vi "SetupAquisitionParameters.vi"(5 "error in":errorcluster) -> (19 "error out":errorcluster)   [LabVIEW 2010]
uses:
  lib/atmcd32d.llb/Error Code Enum typedef.ctl
  lib/atmcd32d.llb/AcquisitionMode_mode typedef.ctl
  lib/atmcd32d.llb/TriggerMode_mode typedef.ctl
  lib/atmcd32d.llb/ReadMode_mode typedef.ctl
  lib/atmcd32d.llb/OutputAmplifier_type typedef.ctl
  lib/atmcd32d.llb/Spool_method typedef.ctl
  Variables/GlobalGetSetMeasurementType.vi
  Variables/GlobalSetGetConfigureCamera.vi
  Variables/GlobalSetGetPixelOfRoi.vi
  Variables/GlobalGetTimingsFromCamera.vi
  lib/atmcd32d.llb/Shutter_mode typedef.ctl
  lib/atmcd32d.llb/Shutter_type typedef.ctl
  lib/atmcd32d.llb/EMGainMode_mode typedef.ctl
panel:
  out "keepCleanTime":sgl
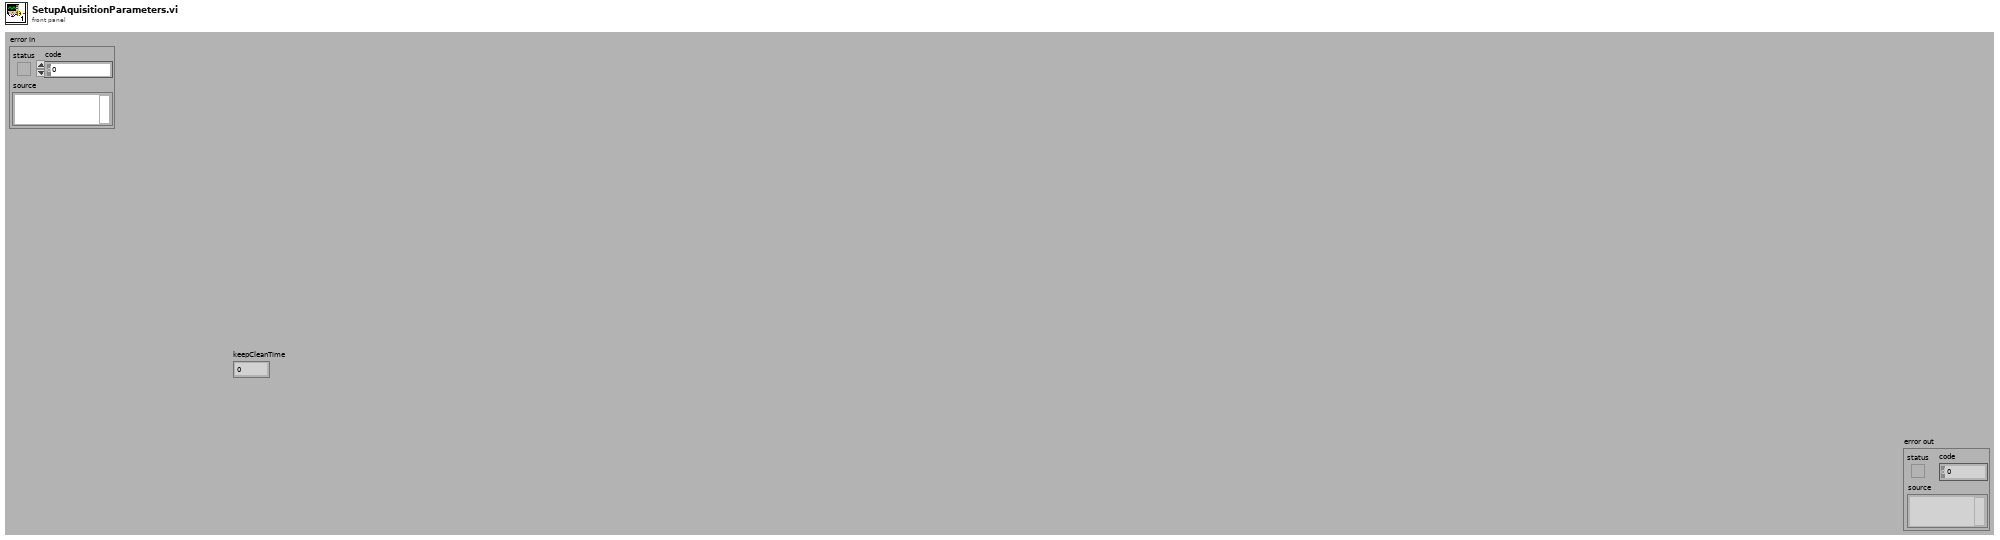
[diagram p1: front panel]
types:
  T1 = cluster{"exposure":sgl, "accumulate":sgl, "kinetic":sgl}
  T2 = typedef "Error Code Enum typedef.ctl" = enum32{"N/A (0)", "DRV_ERROR_CODES", "DRV_SUCCESS", "DRV_VXDNOTINSTALLED", "DRV_ERROR_SCAN", "DRV_ERROR_CHECK_SUM", "DRV_ERROR_FILELOAD", "DRV_UNKNOWN_FUNC", "DRV_ERROR_VXD_INIT", "DRV_ERROR_ADDRESS", "DRV_ERROR_PAGELOCK", "DRV_ERROR_PAGEUNLOCK", "DRV_ERROR_BOARDTEST", "DRV_ERROR_ACK", "DRV_ERROR_UP_FIFO", "DRV_ERROR_PATTERN", "N/A (16)", "DRV_ACQUISITION_ERRORS", "DRV_ACQ_BUFFER", "DRV_ACQ_DOWNFIFO_FULL", "DRV_PROC_UNKONWN_INSTRUCTION", "DRV_ILLEGAL_OP_CODE", "DRV_KINETIC_TIME_NOT_MET", "DRV_ACCUM_TIME_NOT_MET", "DRV_NO_NEW_DATA", "N/A (25)", "DRV_SPOOLERROR", "N/A (27)", "N/A (28)", "N/A (29)", "N/A (30)", "N/A (31)", "N/A (32)", "DRV_TEMPERATURE_CODES", "DRV_TEMPERATURE_OFF", "DRV_TEMPERATURE_NOT_STABILIZED", "DRV_TEMPERATURE_STABILIZED", "DRV_TEMPERATURE_NOT_REACHED", "DRV_TEMPERATURE_OUT_RANGE", "DRV_TEMPERATURE_NOT_SUPPORTED", "DRV_TEMPERATURE_DRIFT", "N/A (41)", "N/A (42)", "N/A (43)", "N/A (44)", "N/A (45)", "N/A (46)", "N/A (47)", "N/A (48)", "DRV_GENERAL_ERRORS", "DRV_INVALID_AUX", "DRV_COF_NOTLOADED", "DRV_FPGAPROG", "DRV_FLEXERROR", "DRV_GPIBERROR", "N/A (55)", "N/A (56)", "N/A (57)", "N/A (58)", "N/A (59)", "N/A (60)", "N/A (61)", "N/A (62)", "N/A (63)", "DRV_DATATYPE", "DRV_DRIVER_ERRORS", "DRV_P1INVALID", "DRV_P2INVALID", "DRV_P3INVALID", "DRV_P4INVALID", "DRV_INIERROR", "DRV_COFERROR", "DRV_ACQUIRING", "DRV_IDLE", "DRV_TEMPCYCLE", "DRV_NOT_INITIALIZED", "DRV_P5INVALID", "DRV_P6INVALID", "DRV_INVALID_MODE", "DRV_INVALID_FILTER", "DRV_I2CERRORS", "DRV_I2CDEVNOTFOUND", "DRV_I2CTIMEOUT", "DRV_P7INVALID", "N/A (84)", "N/A (85)", "N/A (86)", "N/A (87)", "N/A (88)", "N/A (89)", "DRV_IOCERROR", "DRV_VRMVERSIONERROR"}
  T3 = typedef "EMGainMode_mode typedef.ctl" = enum16{"8-bit", "12-bit", "Linear", "Real"}
  T4 = typedef "AcquisitionMode_mode typedef.ctl" = enum16{"Reserved (0)", "Single Scan", "Accumulate", "Kinetics", "Fast Kinetics", "Run Till Abort", "Reserved (6)", "Reserved (7)", "Reserved (8)", "Time Delayed Integration"}
  T5 = typedef "Spool_method typedef.ctl" = enum16{"32-bit", "Depends", "16-bit", "Multiple Directory", "Spool to RAM disk", "16-bit FITS", "SIF", "16-buit TIFF", "Multiple Directory Compressed"}
  T6 = typedef "OutputAmplifier_type typedef.ctl" = enum16{"Standard EMCCD gain register", "Conventional CCD register"}
  T7 = typedef "ReadMode_mode typedef.ctl" = enum16{"Full Vertical Binning", "Multi-Track", "Random-Track", "Single-Track", "Image"}
  T8 = typedef "TriggerMode_mode typedef.ctl" = enum16{"Internal", "External", "N/A (2)", "N/A (3)", "N/A (4)", "N/A (5)", "External Start"}
  T9 = typedef "Shutter_type typedef.ctl" = enum16{"TTL Low", "TTL High"}
  T10 = typedef "Shutter_mode typedef.ctl" = enum16{"Auto", "Open", "Close"}
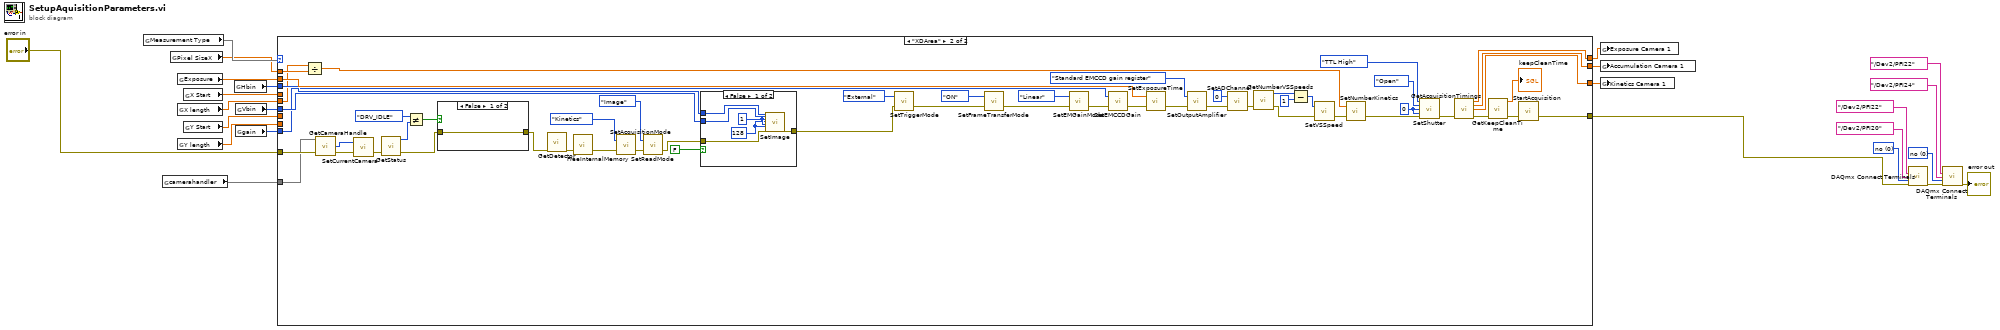
[diagram p0: block diagram]
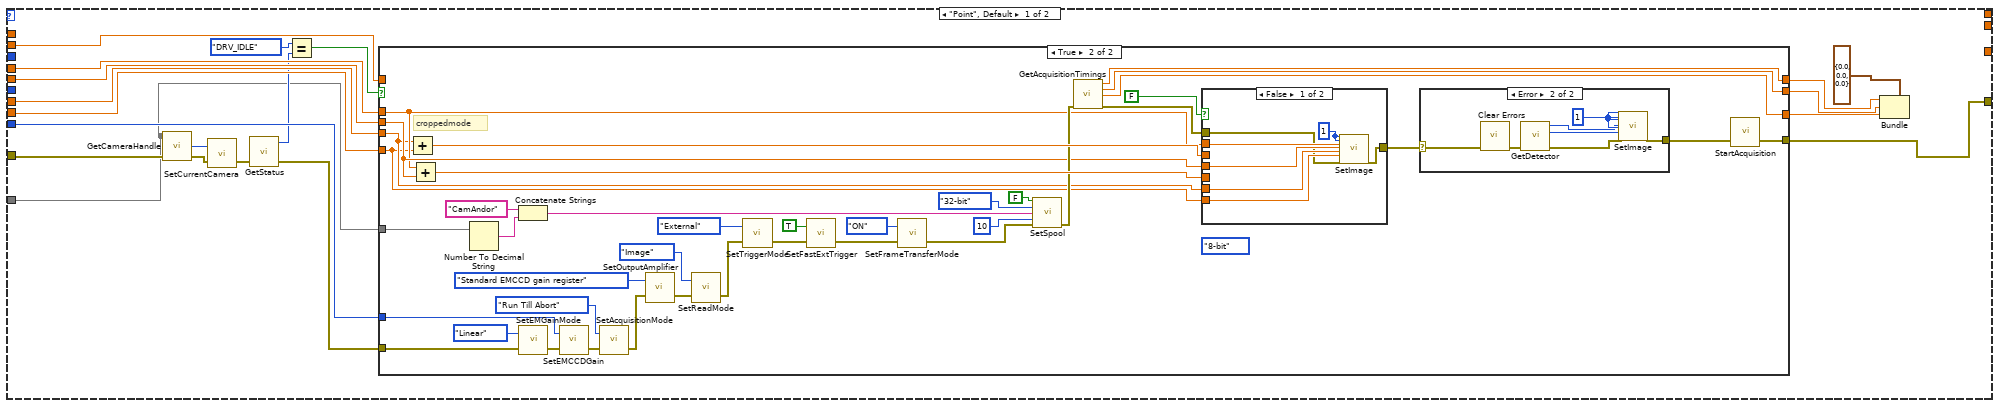
[diagram p2: hidden frame]
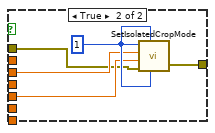
[diagram p4: hidden frame]
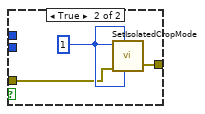
[diagram p6: hidden frame]
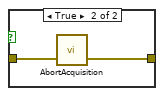
[diagram p7: hidden frame]
diagram:
  w24 = 0 items=["no", "yes"] ("invert polarity")
  w20 = 0 items=["no", "yes"] ("invert polarity")
  n1 = global read "GlobalGetSetMeasurementType.vi" "Measurement Type"() -> (w14)
  n2 = global read "GlobalSetGetConfigureCamera.vi" "camerahandler"() -> (w1)
  n3 = global read "GlobalSetGetPixelOfRoi.vi" "Pixel SizeX"() -> (w10:dbl)
  n4 = global read "GlobalSetGetConfigureCamera.vi" "Exposure"() -> (w13:sgl)
  n5 = global read "GlobalSetGetPixelOfRoi.vi" "X length"() -> (w9:dbl)
  n6 = global read "GlobalSetGetPixelOfRoi.vi" "Y length"() -> (w6:dbl)
  n7 = global read "GlobalSetGetPixelOfRoi.vi" "X Start"() -> (w8:dbl)
  n8 = global read "GlobalSetGetPixelOfRoi.vi" "Y Start"() -> (w7:dbl)
  n9 = global read "GlobalSetGetConfigureCamera.vi" "Hbin"() -> (w11:i32)
  n10 = global read "GlobalSetGetConfigureCamera.vi" "Vbin"() -> (w12:i32)
  n11 = global read "GlobalSetGetConfigureCamera.vi" "gain"() -> (w4:i32)
  n12 = case shown="\"XDArea\"" w14 {
    tunnel: "error in" -> [w44 w158]
    tunnel: w13 -> [w43 w156]
    tunnel: [w42 w157] -> w16
    tunnel: w11 -> [_ w155]
    tunnel: w12 -> [_ w154]
    tunnel: w10 -> [_ w153]
    tunnel: w9 -> [w41 w152]
    tunnel: w8 -> [w40 _]
    tunnel: w7 -> [w39 _]
    tunnel: w6 -> [w38 _]
    tunnel: [_ w108] -> w5
    tunnel: w4 -> [w37 w151]
    tunnel: [_ w107] -> w3
    tunnel: [_ w106] -> w2
    tunnel: w1 -> [w25 w105]
    frame "Point", Default {
      n13 = call "GetCameraHandle.vi"("error in (no error)"=w44, "cameraIndex"=w25) -> ("error out"=w35:errorcluster, "cameraHandle"=w36:i32)  [unwired: 1 in, 1 out]
      n14 = call "SetCurrentCamera.vi"("error in (no error)"=w35, "cameraHandle"=w36) -> ("error out"=w34:errorcluster)  [unwired: 1 out]
      n15 = call "GetStatus.vi"("error in (no error)"=w34) -> ("error out"=w33:errorcluster, "status"=w31:T2)  [unwired: 2 in, 1 out]
      n16 = Equal?(x=Error_Code_Enum_typedef."DRV_IDLE" ("status"), y=w31) -> (x = y?=w30:bool)
      n17 = case shown="True" w30 {
        tunnel: [w45 w81] -> w42
        tunnel: w33 -> [w45 w46]
        tunnel: w25 -> [_ w78]
        tunnel: w43 -> [_ _]
        tunnel: [_ w69] -> w29
        tunnel: [_ w68] -> w28
        tunnel: [_ w67] -> w27
        tunnel: w41 -> [_ w55]
        tunnel: w40 -> [_ w54]
        tunnel: w39 -> [_ w53]
        tunnel: w38 -> [_ w52]
        tunnel: w37 -> [_ w47]
        frame False {
        }
        frame True {
          (unwired) EMGainMode_mode_typedef."8-bit" ("mode")
          # "croppedmode"
          n18 = Add(x=w53, y=w52) -> (x+y=w74:dbl)
          n19 = Add(x=w54, y=w55) -> (x+y=w73:dbl)
          n20 = Number To Decimal String(number=w78) -> (decimal integer string=w79:string)  [unwired: 1 in]
          n21 = Concatenate Strings("CamAndor" ("string"), w79) -> (w77:string)
          n22 = call "SetEMGainMode.vi"("error in (no error)"=w46, "mode"=EMGainMode_mode_typedef."Linear") -> ("error out"=w50:errorcluster)  [unwired: 1 out]
          n23 = call "SetEMCCDGain.vi"("error in (no error)"=w50, "gain"=w47) -> ("error out"=w49:errorcluster)  [unwired: 1 out]
          n24 = call "SetAcquisitionMode.vi"("error in (no error)"=w49, "mode"=AcquisitionMode_mode_typedef."Run Till Abort") -> ("error out"=w76:errorcluster)  [unwired: 1 out]
          n25 = call "SetOutputAmplifier.vi"("error in (no error)"=w76, "type"=OutputAmplifier_type_typedef."Standard EMCCD gain register") -> ("error out"=w56:errorcluster)  [unwired: 1 out]
          n26 = call "SetReadMode.vi"("error in (no error)"=w56, "mode"=ReadMode_mode_typedef."Image") -> ("error out"=w83:errorcluster)  [unwired: 1 out]
          n27 = call "SetTriggerMode.vi"("error in (no error)"=w83, "mode"=TriggerMode_mode_typedef."External") -> ("error out"=w82:errorcluster)  [unwired: 1 out]
          n28 = call "SetFastExtTrigger.vi"("error in (no error)"=w82, "mode"=TRUE) -> ("error out"=w84:errorcluster)  [unwired: 1 out]
          n29 = call "SetFrameTransferMode.vi"("error in (no error)"=w84, "mode"=enum16{"OFF", "ON"}."ON") -> ("error out"=w51:errorcluster)  [unwired: 1 out]
          n30 = call "SetSpool.vi"("active"=FALSE, "method"=Spool_method_typedef."32-bit", "name"=w77, "framebuffersize (10)"=10, "error in (no error)"=w51) -> ("error out"=w70:errorcluster)  [unwired: 9 in, 1 out]
          n31 = call "GetAcquisitionTimings.vi"("error in (no error)"=w70) -> ("exposure"=w69:sgl, "accumulate"=w68:sgl, "kinetic"=w67:sgl, "error out"=w72:errorcluster)  [unwired: 10 in, 1 out]
          n32 = case shown="False" FALSE {
            tunnel: w74 -> [_ w95]
            tunnel: w73 -> [_ w94]
            tunnel: w72 -> [w87 w93]
            tunnel: [w86 w92] -> w71
            tunnel: w54 -> [w90 _]
            tunnel: w53 -> [w89 _]
            tunnel: w55 -> [w91 _]
            tunnel: w52 -> [w88 _]
            frame False {
              w85 = 1
              n33 = call "SetImage.vi"("hbin"=w85, "vbin"=w85, "hstart"=w90, "hend"=w91, "vstart"=w89, "vend"=w88, "error in (no error)"=w87) -> ("error out"=w86:errorcluster)  [unwired: 19 in, 1 out]
            }
            frame True {
              w96 = 1 ("hbin")
              n34 = call "SetIsolatedCropMode.vi"("hbin"=w96, "vbin"=w96, "error in (no error)"=w93, "cropWidth"=w94, "cropHeight"=w95, "active"=w96) -> ("error out"=w92:errorcluster)  [unwired: 1 out]
            }
          }
          n35 = case shown="Error" w71 {
            selector: w71 -> [w97 w100]
            tunnel: [w97 w104] -> w75
            frame No Error {
            }
            frame Error {
              w103 = 1
              n36 = call <vilib>:"Clear Errors.vi"("error in (no error)"=w100) -> ("error out"=w101:errorcluster)  [unwired: 6 in]
              n37 = call "GetDetector.vi"("error in (no error)"=w101) -> ("error out"=w102:errorcluster, "ypixels"=w98:i32, "xpixels"=w99:i32)  [unwired: 3 in, 1 out]
              n38 = call "SetImage.vi"("hbin"=w103, "vbin"=w103, "hstart"=w103, "hend"=w99, "vstart"=w103, "vend"=w98, "error in (no error)"=w102) -> ("error out"=w104:errorcluster)  [unwired: 19 in, 1 out]
            }
          }
          n39 = call "StartAcquisition.vi"("error in (no error)"=w75) -> ("error out"=w81:errorcluster)  [unwired: 1 in, 1 out]
        }
      }
      n40 = Bundle(cluster=T1 {"exposure"=0.0, "accumulate"=0.0, "kinetic"=0.0} ("out 2"), "exposure"=w29, "accumulate"=w28, "kinetic"=w27) -> ()  [unwired: 1 out]
    }
    frame "XDArea" {
      w117 = 0 ("closingtime")
      n41 = Divide(x=w152, y=w153) -> (x/y=w136:dbl)
      n42 = call "GetCameraHandle.vi"("error in (no error)"=w158, "cameraIndex"=w105) -> ("error out"=w149:errorcluster, "cameraHandle"=w150:i32)  [unwired: 1 in, 1 out]
      n43 = call "SetCurrentCamera.vi"("error in (no error)"=w149, "cameraHandle"=w150) -> ("error out"=w148:errorcluster)  [unwired: 1 out]
      n44 = call "GetStatus.vi"("error in (no error)"=w148) -> ("error out"=w147:errorcluster, "status"=w145:T2)  [unwired: 2 in, 1 out]
      n45 = Not Equal?(x=Error_Code_Enum_typedef."DRV_IDLE" ("status"), y=w145) -> (x != y?=w144:bool)
      n46 = case shown="False" w144 {
        tunnel: w147 -> [w168 w170]
        tunnel: [w168 w169] -> w134
        frame False {
        }
        frame True {
          n47 = call "AbortAcquisition.vi"("error in (no error)"=w170) -> ("error out"=w169:errorcluster)  [unwired: 1 in, 1 out]
        }
      }
      n48 = call "GetDetector.vi"("error in (no error)"=w134) -> ("error out"=w135:errorcluster)  [unwired: 3 in, 3 out]
      n49 = call "FreeInternalMemory.vi"("error in (no error)"=w135) -> ("error out"=w137:errorcluster)  [unwired: 1 in, 1 out]
      n50 = call "SetAcquisitionMode.vi"("error in (no error)"=w137, "mode"=AcquisitionMode_mode_typedef."Kinetics") -> ("error out"=w133:errorcluster)  [unwired: 1 out]
      n51 = call "SetReadMode.vi"("error in (no error)"=w133, "mode"=ReadMode_mode_typedef."Image") -> ("error out"=w132:errorcluster)  [unwired: 1 out]
      n52 = case shown="False" FALSE {
        tunnel: w132 -> [w164 w166]
        tunnel: [w163 w165] -> w118
        tunnel: w155 -> [w160 _]
        tunnel: w154 -> [w159 _]
        frame False {
          w161 = 128 ("hend")
          w162 = 1 ("hstart")
          n53 = call "SetImage.vi"("hbin"=w160, "vbin"=w159, "hstart"=w162, "hend"=w161, "vstart"=w162, "vend"=w161, "error in (no error)"=w164) -> ("error out"=w163:errorcluster)  [unwired: 19 in, 1 out]
        }
        frame True {
          w167 = 1 ("hbin")
          n54 = call "SetIsolatedCropMode.vi"("hbin"=w167, "vbin"=w167, "error in (no error)"=w166, "active"=w167) -> ("error out"=w165:errorcluster)  [unwired: 2 in, 1 out]
        }
      }
      n55 = call "SetTriggerMode.vi"("error in (no error)"=w118, "mode"=TriggerMode_mode_typedef."External") -> ("error out"=w131:errorcluster)  [unwired: 1 out]
      n56 = call "SetFrameTransferMode.vi"("error in (no error)"=w131, "mode"=enum16{"OFF", "ON"}."ON") -> ("error out"=w109:errorcluster)  [unwired: 1 out]
      n57 = call "SetEMGainMode.vi"("error in (no error)"=w109, "mode"=EMGainMode_mode_typedef."Linear") -> ("error out"=w114:errorcluster)  [unwired: 1 out]
      n58 = call "SetEMCCDGain.vi"("error in (no error)"=w114, "gain"=w151) -> ("error out"=w113:errorcluster)  [unwired: 1 out]
      n59 = call "SetExposureTime.vi"("error in (no error)"=w113, "time"=w156) -> ("error out"=w112:errorcluster)  [unwired: 1 out]
      n60 = call "SetOutputAmplifier.vi"("error in (no error)"=w112, "type"=OutputAmplifier_type_typedef."Standard EMCCD gain register") -> ("error out"=w111:errorcluster)  [unwired: 1 out]
      n61 = call "SetADChannel.vi"("error in (no error)"=w111, "channel"=0) -> ("error out"=w129:errorcluster)  [unwired: 1 out]
      n62 = call "GetNumberVSSpeeds.vi"("error in (no error)"=w129) -> ("error out"=w128:errorcluster, "number"=w127:i32)  [unwired: 2 in, 1 out]
      n63 = Subtract(x=w127, y=1) -> (x-y=w125:i32)
      n64 = call "SetVSSpeed.vi"("error in (no error)"=w128, "index"=w125) -> ("error out"=w124:errorcluster)  [unwired: 1 out]
      n65 = call "SetNumberKinetics.vi"("error in (no error)"=w124, "number"=w136) -> ("error out"=w123:errorcluster)  [unwired: 1 out]
      n66 = call "SetShutter.vi"("type"=Shutter_type_typedef."TTL High", "mode"=Shutter_mode_typedef."Open", "closingtime"=w117, "openingtime"=w117, "error in (no error)"=w123) -> ("error out"=w121:errorcluster)  [unwired: 9 in, 1 out]
      n67 = call "GetAcquisitionTimings.vi"("error in (no error)"=w121) -> ("exposure"=w106:sgl, "accumulate"=w107:sgl, "kinetic"=w108:sgl, "error out"=w120:errorcluster)  [unwired: 10 in, 1 out]
      n68 = call "GetKeepCleanTime.vi"("error in (no error)"=w120) -> ("error out"=w119:errorcluster, "keepCleanTime"=→"keepCleanTime":sgl)  [unwired: 4 in, 1 out]
      n69 = call "StartAcquisition.vi"("error in (no error)"=w119) -> ("error out"=w157:errorcluster)  [unwired: 1 in, 1 out]
    }
  }
  n70 = global write "GlobalGetTimingsFromCamera.vi" "Exposure Camera 1"(w2) -> ()
  n71 = global write "GlobalGetTimingsFromCamera.vi" "Accumulation Camera 1"(w3) -> ()
  n72 = global write "GlobalGetTimingsFromCamera.vi" "Kinetics Camera 1"(w5) -> ()
  n73 = call <vilib>:"DAQmx Connect Terminals.vi"("source terminal"=tag "/Dev2/PFI22", "destination terminal"=tag "/Dev2/PFI20", "invert polarity"=w20, "error in"=w16) -> ("error out"=w21:errorcluster)  [unwired: 11 in]
  n74 = call <vilib>:"DAQmx Connect Terminals.vi"("source terminal"=tag "/Dev2/PFI22", "destination terminal"=tag "/Dev2/PFI24", "invert polarity"=w24, "error in"=w21) -> ("error out"=→"error out":errorcluster)  [unwired: 11 in]
